vi "Draw Image From File.vi"(8 "error in":errorcluster, 11 "Image Path In":path) -> (0 "error out":errorcluster, 3 "Picture Out":picture)   [LabVIEW 2016, in "MetaDataObj.lvclass"]
uses:
  <resource>/dialog/NewProjectWizard/MetaDataObj/MetaDataObj.lvclass
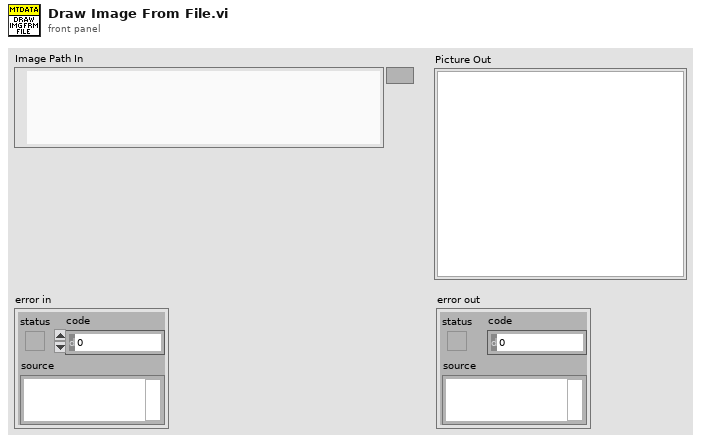
[diagram p1: front panel]
types:
  T1 = typedef "imagedata.ctl" = cluster{"image type":i32, "image depth":i32, "image":u8[], "mask":u8[], "colors":u32[], "Rectangle":cluster{"left":i16, "top":i16, "right":i16, "bottom":i16}}
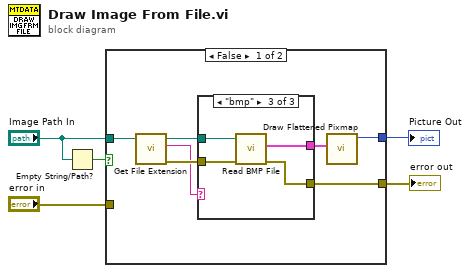
[diagram p0: block diagram]
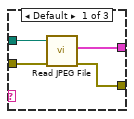
[diagram p2: hidden frame]
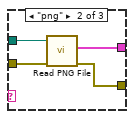
[diagram p3: hidden frame]
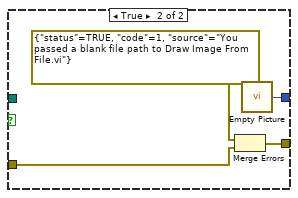
[diagram p4: hidden frame]
diagram:
  n1 = Empty String/Path?(string/path="Image Path In") -> (empty?=w4:bool)
  n2 = case shown="False" w4 {
    tunnel: "Image Path In" -> [w6 _]
    tunnel: [w11 w28] -> w3
    tunnel: [w10 w27] -> w2
    tunnel: "error in" -> [_ w26]
    frame False {
      n3 = call <vilib>:"Get File Extension.vi"("file"=w6) -> ("error out"=w9:errorcluster, "lowercase file extension"=w8:string, "dup file"=w7:path)  [unwired: 6 in, 2 out]
      n4 = case shown="\"bmp\"" w8 {
        tunnel: w7 -> [w16 w19 w24]
        tunnel: [w15 w20 w23] -> w12
        tunnel: [w13 w18 w21] -> w10
        tunnel: w9 -> [w14 w17 w22]
        frame Default {
          n5 = call <vilib>:"Read JPEG File.vi"("error in (no error)"=w14, "path to JPEG file"=w16) -> ("error out"=w13:errorcluster, "image data"=w15:T1)  [unwired: 7 in, 1 out]
        }
        frame "png" {
          n6 = call <vilib>:"Read PNG File.vi"("error in (no error)"=w17, "path to PNG file"=w19) -> ("error out"=w18:errorcluster, "image data"=w20:T1)  [unwired: 7 in, 1 out]
        }
        frame "bmp" {
          n7 = call <vilib>:"Read BMP File.vi"("error in (no error)"=w22, "path to BMP file"=w24) -> ("error out"=w21:errorcluster, "image data"=w23:T1)  [unwired: 7 in, 1 out]
        }
      }
      n8 = call <vilib>:"Draw Flattened Pixmap.vi"("image data"=w12) -> ("new picture"=w11:picture)  [unwired: 8 in]
    }
    frame True {
      n9 = Merge Errors(errorcluster {"status"=TRUE, "code"=1, "source"="You passed a blank file path to Draw Image From File.vi"} ("error in"), w26) -> (w27:errorcluster)
      n10 = call "Empty Picture"() -> ("empty picture"=w28:picture)
    }
  }
  "Picture Out" <- w3
  "error out" <- w2
